vi "Displayed Row Calc MCL.vi"(8 "Coords.Vertical":i32, 9 "Tree.Position:Top":i32, 10 "TopLeft.Row":i32, 11 "Constant Sizes":T1) -> (2 "Pixels from top of row":i32, 3 "Displayed Row":i32)   [LabVIEW 2020, in "BetterDragAndDrop.lvlib" / "BetterBoxHandle.lvclass"]
uses:
  Classes/BetterBoxHandle/BetterBoxHandle.lvclass
  Classes/BetterHandle/Pixel Constants.ctl
  BetterDragAndDrop.lvlib
  Classes/BetterHandle/BetterHandle.lvclass
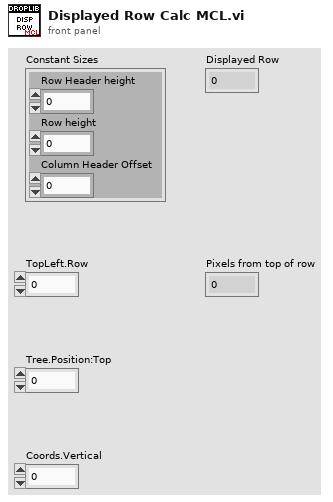
[diagram p1: front panel]
types:
  T1 = typedef "BetterDragAndDrop.lvlib/BetterHandle.lvclass/Pixel Constants.ctl" = cluster{"Row Header height":i32, "Row height":i32, "Column Header Offset":i32}
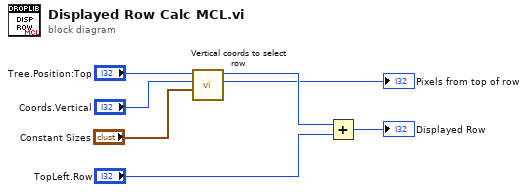
[diagram p0: block diagram]
diagram:
  n1 = call "Vertical coords to select row.vi"("Constant Sizes"="Constant Sizes", "Coords.Vertical"="Coords.Vertical", "Tree.Position:Top"="Tree.Position:Top") -> ("Pixels from top of row"=→"Pixels from top of row":i32, "Displayed Row"=w2:i32)  [unwired: 7 in]
  n2 = Add(x=w2, y="TopLeft.Row") -> (x+y=→"Displayed Row":i32)
